vi "CRYCalc group delay.vi"(9 "Smoothing Width":i32, 11 "Curve in":T1={"Name"="", "Curve"=[], "X data"=1, "Y data"=1, "Z data"=1, "X axis"=0, "Y axis"=1, "Z axis"=1, "X unit"="Hz", "Y unit"="", "Z unit"="deg.", "X dB ref"=1.0, "Y dB ref"=1.0, "Z dB ref"=1.0, "single val"=FALSE, "protected"=FALSE, "display X"=TRUE, "display Y"=TRUE, "display Z"=TRUE, "Test Info"="", "Step No."=0, "Plot Settings"={"Color"=0, "Interpolation"=0, "Point Style"=0, "Line Style"=0, "Point Color"=0, "Line Width"=0, "Bar Plot Style"=0, "Fill To"=0}, "AutoProtect"=FALSE} {"Z data" items=["dB", "Lin"]; "X data" items=["dB", "Lin"]; "Y data" items=["dB", "Lin"]; "Z dB ref" format="%.1f"; "Z axis" items=["Log", "Lin"]; "X dB ref" format="%.1f"; "X axis" items=["Log", "Lin"]; "Y axis" items=["Log", "Lin"]; "Y dB ref" format="%.1f"; "Curve"."z" format="%.2f"; "Curve"."y" format="%.2f"; "Curve"."x" format="%.2f"}) -> (3 "Curve out":T1={"Name"="", "Curve"=[], "X data"=1, "Y data"=1, "Z data"=1, "X axis"=0, "Y axis"=1, "Z axis"=1, "X unit"="Hz", "Y unit"="", "Z unit"="deg.", "X dB ref"=1.0, "Y dB ref"=1.0, "Z dB ref"=1.0, "single val"=FALSE, "protected"=FALSE, "display X"=TRUE, "display Y"=TRUE, "display Z"=TRUE, "Test Info"="", "Step No."=0, "Plot Settings"={"Color"=0, "Interpolation"=0, "Point Style"=0, "Line Style"=0, "Point Color"=0, "Line Width"=0, "Bar Plot Style"=0, "Fill To"=0}, "AutoProtect"=FALSE} {"Z data" items=["dB", "Lin"]; "X data" items=["dB", "Lin"]; "Y data" items=["dB", "Lin"]; "Z dB ref" format="%.1f"; "Z axis" items=["Log", "Lin"]; "X dB ref" format="%.1f"; "X axis" items=["Log", "Lin"]; "Y axis" items=["Log", "Lin"]; "Y dB ref" format="%.1f"; "Curve"."z" format="%.2f"; "Curve"."y" format="%.2f"; "Curve"."x" format="%.2f"})   [LabVIEW 2013]
uses:
  Typedef Control/CRYData Cluster.ctl
  <vilib>/Analysis/NI_AALPro.lvlib
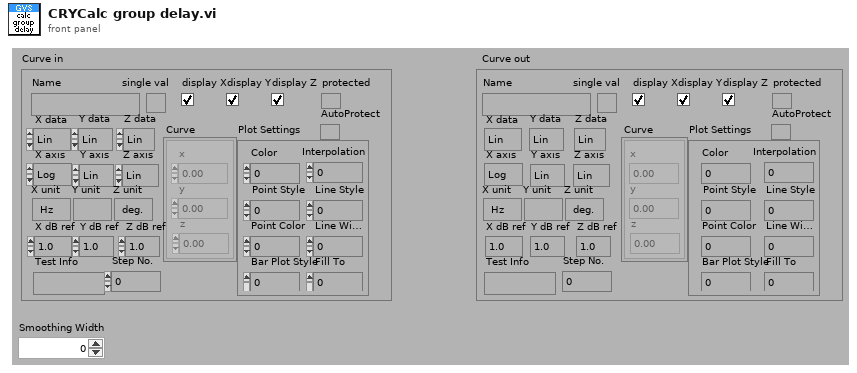
[diagram p1: front panel]
types:
  T1 = typedef "CRYData Cluster.ctl" = cluster{"Name":string, "Curve":cluster{"x":dbl, "y":dbl, "z":dbl}[], "X data":u16, "Y data":u16, "Z data":u16, "X axis":u16, "Y axis":u16, "Z axis":u16, "X unit":string, "Y unit":string, "Z unit":string, "X dB ref":dbl, "Y dB ref":dbl, "Z dB ref":dbl, "single val":bool, "protected":bool, "display X":bool, "display Y":bool, "display Z":bool, "Test Info":string, "Step No.":i32, "Plot Settings":cluster{"Color":u32, "Interpolation":u8, "Point Style":u8, "Line Style":u8, "Point Color":u32, "Line Width":u8, "Bar Plot Style":u8, "Fill To":i16}, "AutoProtect":bool}
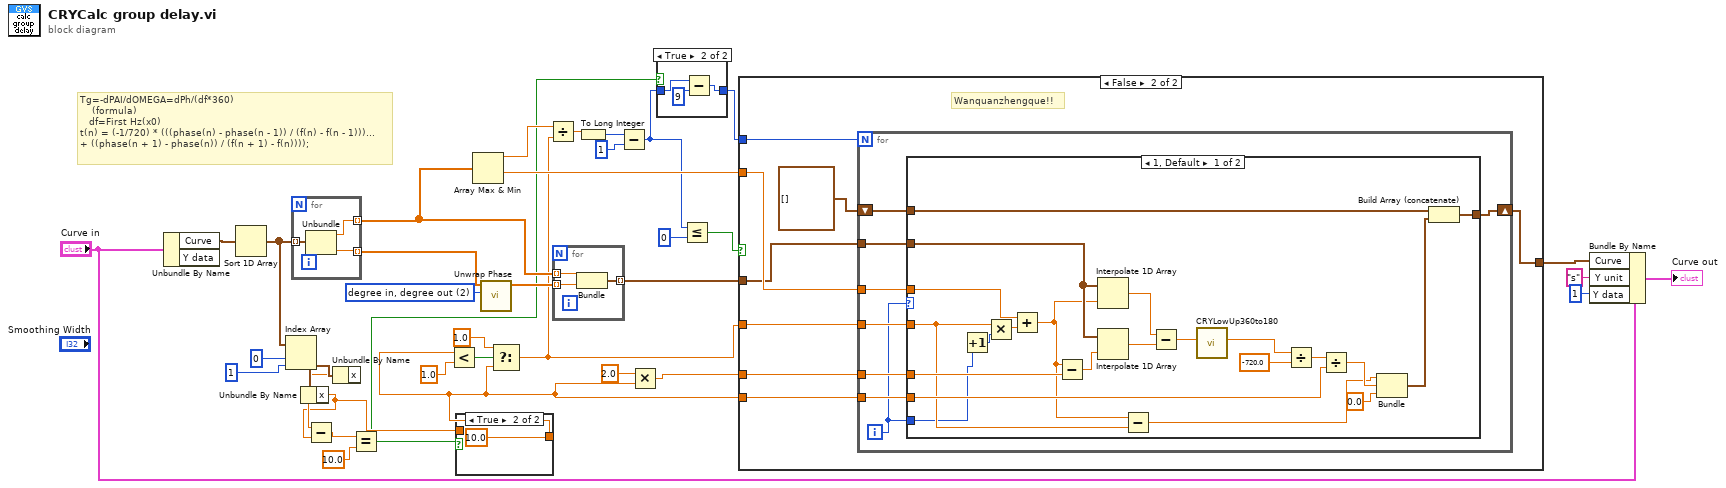
[diagram p0: block diagram]
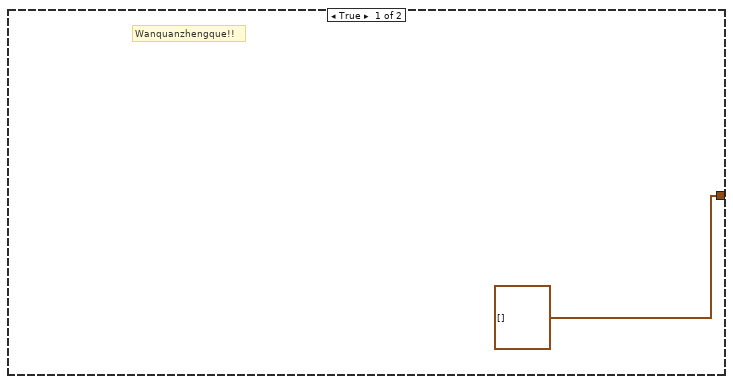
[diagram p4: hidden frame]
diagram:
  w24 = 2 items=["radian in, radian out", "radian in, degree out", "degree in, degree out", "degree in, radian out"] ("phase unit")
  # "Tg=-dPAI/dOMEGA=dPh/(df*360)\n    (formula)\n   df=First Hz(x0)\nt(n) = (-1/720) * (((phase(n) - phase(n - 1)) / (f(n) - f(n - 1)))...\n+ ((phase(n + 1) - phase(n)) / (f(n + 1) - f(n))));"
  n1 = Unbundle By Name("Curve in") -> ("Curve"=w28:cluster{"x":dbl, "y":dbl, "z":dbl}[])  [unwired: 1 out]
  n2 = Sort 1D Array(array=w28) -> (sorted array=w26:cluster{"x":dbl, "y":dbl, "z":dbl}[])
  n3 = Index Array(array=w26, index #1=0, index #2=1) -> (element #1=w27:cluster{"x":dbl, "y":dbl, "z":dbl}, element #2=w9:cluster{"x":dbl, "y":dbl, "z":dbl})
  n4 = for {
    tunnel: w26 -> [w40] mode=indexing
    tunnel: [w39] -> w22 mode=indexing
    tunnel: [w38] -> w25 mode=indexing
    n5 = Unbundle(w40) -> ("x"=w39:dbl, "z"=w38:dbl)  [unwired: 1 out]
  }
  n6 = Unbundle By Name(w27) -> ("x"=w4:dbl)
  n7 = Unbundle By Name(w9) -> ("x"=w8:dbl)
  n8 = Subtract(x=w8, y=w4) -> (x-y=w7:dbl)
  n9 = Equal?(x=w7, y=10.0) -> (x = y?=w3:bool)
  n10 = case shown="True" w3 {
    tunnel: [w41 10.0] -> w6
    tunnel: w4 -> [w41 _]
    frame False {
    }
    frame True {
    }
  }
  n11 = Less?(x=w6, y=1.0) -> (x < y?=w17:bool)
  n12 = Array Max & Min(array=w22) -> (max value=w37:dbl, min value=w30:dbl)  [unwired: 2 out]
  n13 = call <vilib>:"Unwrap Phase.vi"("phase unit"=w24, "Phase"=w25) -> ("Unwrapped Phase"=w23:dbl[])  [unwired: 8 in, 1 out]
  n14 = Select(t=1.0, s=w17, f=w6) -> (s? t:f=w15:dbl)
  n15 = Divide(x=w37, y=w15) -> (x/y=w36:dbl)
  n16 = for {
    tunnel: w23 -> [w45] mode=indexing
    tunnel: w22 -> [w44] mode=indexing
    tunnel: [w43] -> w21 mode=indexing
    n17 = Bundle("x"=w44, w45) -> (w43:cluster{"x":dbl, dbl})  [unwired: 1 in]
  }
  n18 = To Long Integer(number=w36) -> (32bit integer=w31:i32)
  n19 = Subtract(x=w31, y=1) -> (x-y=w2:i32)
  n20 = Multiply(x=2.0, y=w6) -> (x*y=w13:dbl)
  n21 = case shown="True" w3 {
    tunnel: w2 -> [w46 w48]
    tunnel: [w46 w49] -> w1
    frame False {
    }
    frame True {
      n22 = Subtract(x=w48, y=9) -> (x-y=w49:i32)
    }
  }
  n23 = Less Or Equal?(x=w2, y=0) -> (x <= y?=w20:bool)
  n24 = case shown="False" w20 {
    tunnel: w30 -> [_ w58]
    tunnel: w1 -> [_ w57]
    tunnel: w6 -> [_ w56]
    tunnel: w21 -> [_ w55]
    tunnel: w15 -> [_ w54]
    tunnel: w13 -> [_ w53]
    tunnel: [cluster{dbl, dbl, "y":dbl}[] [] w51] -> w12
    frame True {
      # "Wanquanzhengque!!"
    }
    frame False {
      # "Wanquanzhengque!!"
      n25 = for {
        N: w57 -> [_]
        tunnel: w55 -> [w65]
        tunnel: w58 -> [w66]
        tunnel: w56 -> [w64]
        tunnel: w54 -> [w62]
        tunnel: w53 -> [w63]
        shift-right: [w59] -> w51
        shift-left: cluster{dbl, dbl, "y":dbl}[] [] -> [w60]
        i -> [w61]
        n26 = case shown="1, Default" w61 {
          tunnel: w66 -> [w85 _]
          tunnel: w65 -> [w71 _]
          tunnel: w61 -> [w69 _]
          tunnel: w64 -> [w79 _]
          tunnel: w63 -> [w76 _]
          tunnel: w62 -> [w75 _]
          tunnel: w60 -> [w73 w89]
          tunnel: [w72 w89] -> w59
          frame 1, Default {
            n27 = Increment(x=w69) -> (x+1=w70:i32)
            n28 = Multiply(x=w75, y=w70) -> (x*y=w84:dbl)
            n29 = Add(x=w85, y=w84) -> (x+y=w68:dbl)
            n30 = Subtract(x=w68, y=w76) -> (x-y=w80:dbl)
            n31 = Interpolate 1D Array(1:w68, 2:w71) -> (0:w82:dbl)
            n32 = Interpolate 1D Array(1:w80, 2:w71) -> (0:w81:dbl)
            n33 = Subtract(x=w68, y=w75) -> (x-y=w67:dbl)
            n34 = Subtract(x=w82, y=w81) -> (x-y=w78:dbl)
            n35 = call "CRYLowUp360to180.vi"("Value In"=w78) -> ("Value Out"=w77:dbl)  [unwired: 10 in]
            n36 = Divide(x=w77, y=-720.0) -> (x/y=w87:dbl)
            n37 = Divide(x=w87, y=w79) -> (x/y=w83:dbl)
            n38 = Bundle(w67, w83, "y"=0.0) -> (w74:cluster{dbl, dbl, "y":dbl})  [unwired: 1 out]
            n39 = Build Array (concatenate)(w73, w74) -> (w72:cluster{dbl, dbl, "y":dbl}[])
          }
          frame 0 {
          }
        }
      }
    }
  }
  n40 = Bundle By Name(cluster="Curve in", "Curve"=w12, "Y unit"="s", "Y data"=u16 1) -> (→"Curve out":T1)
